vi "Cross Product.vi"(1 "B":dbl[](array[numeric]), 2 "A":dbl[](array[numeric])) -> (0 "AxB":dbl[](array[numeric]))   [LabVIEW 2016, in "fick-matrix.lvlib"]
uses:
  fick-matrix.lvlib
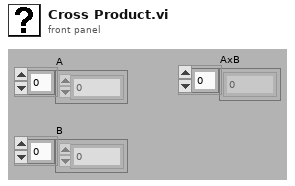
[diagram p1: front panel]
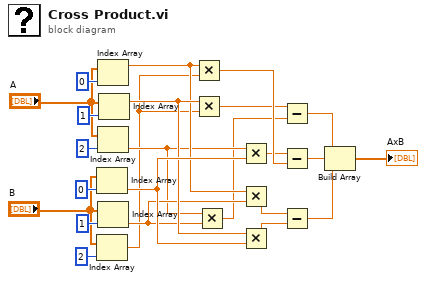
[diagram p0: block diagram]
diagram:
  n1 = Index Array(array="B", index=0) -> (element=w17:dbl)
  n2 = Index Array(array="B", index=2) -> (element=w11:dbl)
  n3 = Index Array(array="A", index=0) -> (element=w14:dbl)
  n4 = Index Array(array="A", index=2) -> (element=w12:dbl)
  n5 = Index Array(array="B", index=1) -> (element=w15:dbl)
  n6 = Index Array(array="A", index=1) -> (element=w16:dbl)
  n7 = Multiply(x=w14, y=w11) -> (x*y=w22:dbl)
  n8 = Multiply(x=w16, y=w11) -> (x*y=w9:dbl)
  n9 = Multiply(x=w12, y=w15) -> (x*y=w10:dbl)
  n10 = Multiply(x=w12, y=w17) -> (x*y=w13:dbl)
  n11 = Multiply(x=w14, y=w15) -> (x*y=w18:dbl)
  n12 = Multiply(x=w16, y=w17) -> (x*y=w19:dbl)
  n13 = Subtract(x=w9, y=w10) -> (x-y=w24:dbl)
  n14 = Subtract(x=w13, y=w22) -> (x-y=w20:dbl)
  n15 = Subtract(x=w18, y=w19) -> (x-y=w21:dbl)
  n16 = Build Array(w24, w20, w21) -> (→"AxB":dbl[])
